vi "Low Level save.vi"(0 "NI_report in":refnum<class "NI_report.lvclass">, 5 "worksheet index (0)":i32, 7 "Array":string[][](array[string]), 9 "Dimming Options":T1, 11 "error in (no error)":errorcluster) -> (4 "NI_report out":refnum<class "NI_report.lvclass">, 6 "position (Excel)":cluster{"row":i32, "column":i32}, 8 "end position":cluster{"row":i32, "column":i32}, 10 "Start position":cluster{"row":i32, "column":i32}, 15 "error out":errorcluster)   [LabVIEW 2016, in "Data Saving.lvlib" / "Excel Saver.lvclass"]
uses:
  Excel Saver.lvclass
  <vilib>/Utility/NIReport.llb/NI_report.lvclass
  Focal Point End Of Line Tester/Controls/Dimming Options.ctl
  <vilib>/addons/_office/excel.llb/Excel Easy Table (str).vi
  <vilib>/Utility/NIReport.llb/Excel/NI_Excel.lvclass
  <vilib>/addons/_office/NI_ReportGenerationToolkit.lvlib
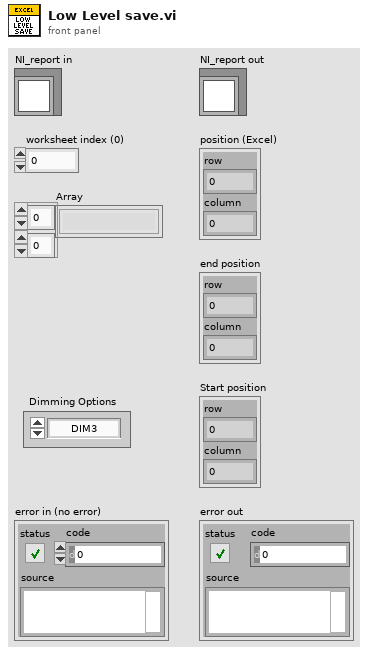
[diagram p1: front panel]
types:
  T1 = typedef "Dimming Options.ctl" = enum16{"DIM3", "DIM2", "DIM1", "NONE"}
  T2 = cluster{"position (Excel)":cluster{"row":i32, "column":i32}, "name (Excel)":string, "bookmark (Word)":string}
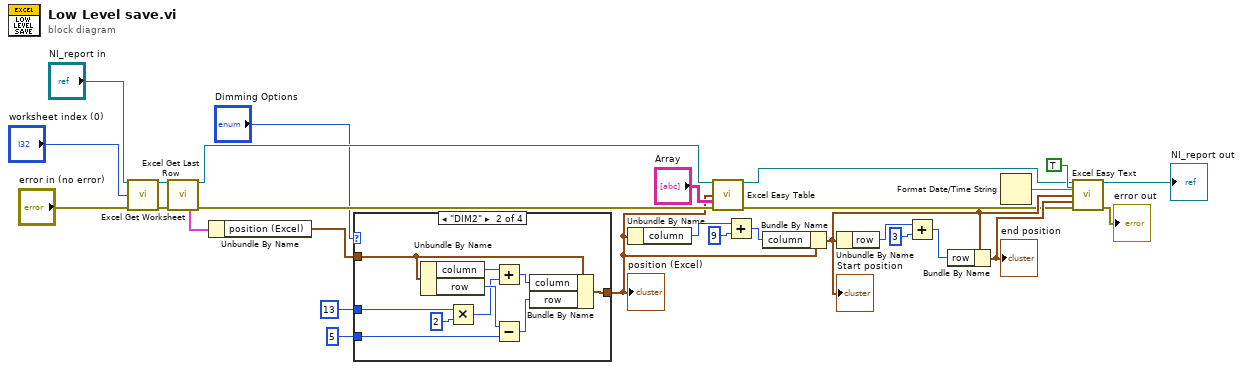
[diagram p0: block diagram]
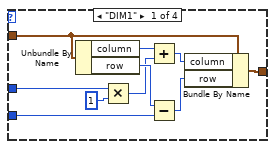
[diagram p2: hidden frame]
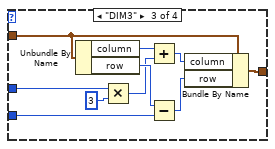
[diagram p3: hidden frame]
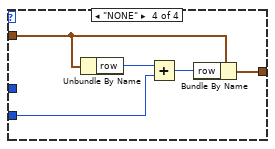
[diagram p4: hidden frame]
diagram:
  n1 = call <vilib>:"Excel Get Worksheet.vi"("report in"="NI_report in", "worksheet index (0)"="worksheet index (0)", "error in (no error)"="error in (no error)") -> ("report out"=w18:refnum<class "NI_report.lvclass">, "error out"=w19:errorcluster)  [unwired: 11 in]
  n2 = call <vilib>:"Excel Get Last Row.vi"("report in"=w18, "error in (no error)"=w19) -> ("report out"=w12:refnum<class "NI_report.lvclass">, "MS Office parameters out"=w11:T2, "error out"=w13:errorcluster)  [unwired: 11 in]
  n3 = Unbundle By Name(w11) -> ("position (Excel)"=w15:cluster{"row":i32, "column":i32})
  n4 = case shown="\"DIM2\"" "Dimming Options" {
    tunnel: w15 -> [w36 w46 w56 w63]
    tunnel: [w35 w45 w55 w62] -> w10
    tunnel: 5 ("y") -> [w33 w43 w53 w59]
    tunnel: 13 ("y") -> [w31 w41 w51 _]
    frame "DIM1" {
      n5 = Unbundle By Name(w36) -> ("column"=w37:i32, "row"=w34:i32)
      n6 = Multiply(x=w31, y=1) -> (x*y=w30:i32)
      n7 = Add(x=w37, y=w30) -> (x+y=w38:i32)
      n8 = Subtract(x=w34, y=w33) -> (x-y=w32:i32)
      n9 = Bundle By Name(cluster=w36, "column"=w38, "row"=w32) -> (w35:cluster{"row":i32, "column":i32})
    }
    frame "DIM2" {
      n10 = Unbundle By Name(w46) -> ("column"=w47:i32, "row"=w44:i32)
      n11 = Multiply(x=w41, y=2) -> (x*y=w40:i32)
      n12 = Add(x=w47, y=w40) -> (x+y=w48:i32)
      n13 = Subtract(x=w44, y=w43) -> (x-y=w42:i32)
      n14 = Bundle By Name(cluster=w46, "column"=w48, "row"=w42) -> (w45:cluster{"row":i32, "column":i32})
    }
    frame "DIM3" {
      n15 = Unbundle By Name(w56) -> ("column"=w57:i32, "row"=w54:i32)
      n16 = Multiply(x=w51, y=3) -> (x*y=w50:i32)
      n17 = Add(x=w57, y=w50) -> (x+y=w58:i32)
      n18 = Subtract(x=w54, y=w53) -> (x-y=w52:i32)
      n19 = Bundle By Name(cluster=w56, "column"=w58, "row"=w52) -> (w55:cluster{"row":i32, "column":i32})
    }
    frame "NONE" {
      n20 = Unbundle By Name(w63) -> ("row"=w60:i32)
      n21 = Add(x=w60, y=w59) -> (x+y=w61:i32)
      n22 = Bundle By Name(cluster=w63, "row"=w61) -> (w62:cluster{"row":i32, "column":i32})
    }
  }
  "position (Excel)" <- w10
  n23 = Unbundle By Name(w10) -> ("column"=w4:i32)
  n24 = call-poly <vilib>:"Excel Easy Table.vi"("report in"=w12, "start (0, 0)"=w10, "text data"="Array", "error in (no error)"=w13) -> ("report out"=w20:refnum<class "NI_report.lvclass">, "error out"=w22:errorcluster)  [unwired: 7 in, 3 out]
  n25 = Add(x=w4, y=9) -> (x+y=w6:i32)
  n26 = Bundle By Name(cluster=w10, "column"=w6) -> (w25:cluster{"row":i32, "column":i32})
  "Start position" <- w25
  n27 = Unbundle By Name(w25) -> ("row"=w7:i32)
  n28 = Add(x=w7, y=3) -> (x+y=w9:i32)
  n29 = Bundle By Name(cluster=w25, "row"=w9) -> (w26:cluster{"row":i32, "column":i32})
  "end position" <- w26
  n30 = Format Date/Time String() -> (date/time string=w24:string)  [unwired: 3 in]
  n31 = call <vilib>:"Excel Easy Text.vi"("report in"=w20, "border? (F)"=TRUE, "text"=w24, "start (-1, -1)"=w25, "end (-1, -1)"=w26, "error in (no error)"=w22) -> ("report out"=→"NI_report out":refnum<class "NI_report.lvclass">, "error out"=→"error out":errorcluster)  [unwired: 5 in, 3 out]
